vi "SpiralSearchForObserver.vi"() -> ()   [LabVIEW 2009, in "DelayGenerator.lvlib"]
uses:
  DelayGenerator.lvlib
  Aerotech/Controls/AerotechTarget.ctl
  Controls/DelayGenerator.ctl
  <vilib>/Utility/file.llb/Write To Spreadsheet File (string).vi
panel:
  out "Equivalent 0 OPD Aerotech":dbl[unit]=0.4973897187765687
  out "Actual Offset (real)":dbl[unit]=-0.9947794375531374
  in  "Tab Control":enum32{"OffSet", "Aerotech Position"}(tab)
  out "Waveform Chart":dbl[unit](graph)=-0.9947794375531374
  out "Aerotech":T1(graph)
  in  "file (use dialog)":path=path "C:/Ohana_Development/Data/Ciel juillet 2010/logOffset120710.txt"
  in  "Central Carriage\nPosition":dbl[unit]=5.4
  in  "longueur":dbl[unit]=0.000128
  out "timeout":bool
  out "AEROTECH.ACTUAL":T2={"Time"=timestamp(3360926630.935375 s since 1904-01-01), "Position"=0.49738967, "Velocity"=2.43882843364851e-08}
  in  "0 OPD Aerotech position at 5.4":dbl[unit]=0.494234
  in  "Manual step Aerotech":dbl[unit]=1.2e-05
  in  "en arrière":bool
  in  "en avant":bool
  in  "Automatic":bool
  in  "Gain":dbl=0.3
  out "amplitude mouvement":dbl[unit]=2.133333333333333e-05
  out "compteur":i32=3565
  in  "+/-1":dbl=-1.0
  out "step Aerotech":dbl[unit]=2.133333333333333e-05
  in  "sens":bool=TRUE
  in  "Unidirectionnel":bool=TRUE
  out "position frange":dbl(slide)=-0.10617897727272729 max=9.49392237e-316 scale=-1.0..1.0
  out "centre spirale":dbl[unit]=0.4973897187765687
  out "Frange":bool=TRUE
  in  "stop":bool
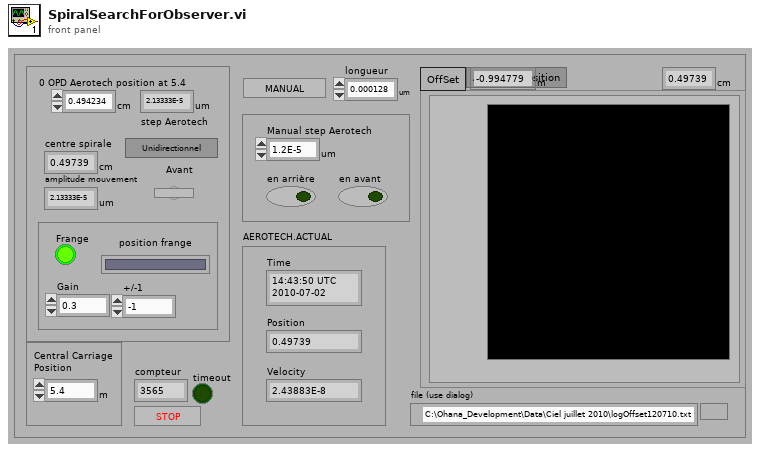
[diagram p1: front panel]
types:
  T1 = cluster{"0 OPD Aerotech position at 5.4":dbl[unit], dbl[unit]}
  T2 = typedef "AerotechTarget.ctl" = cluster{"Time":timestamp, "Position":dbl, "Velocity":dbl}
  T3 = typedef "DelayGenerator.ctl" = cluster{"OpticalPasses":i32}
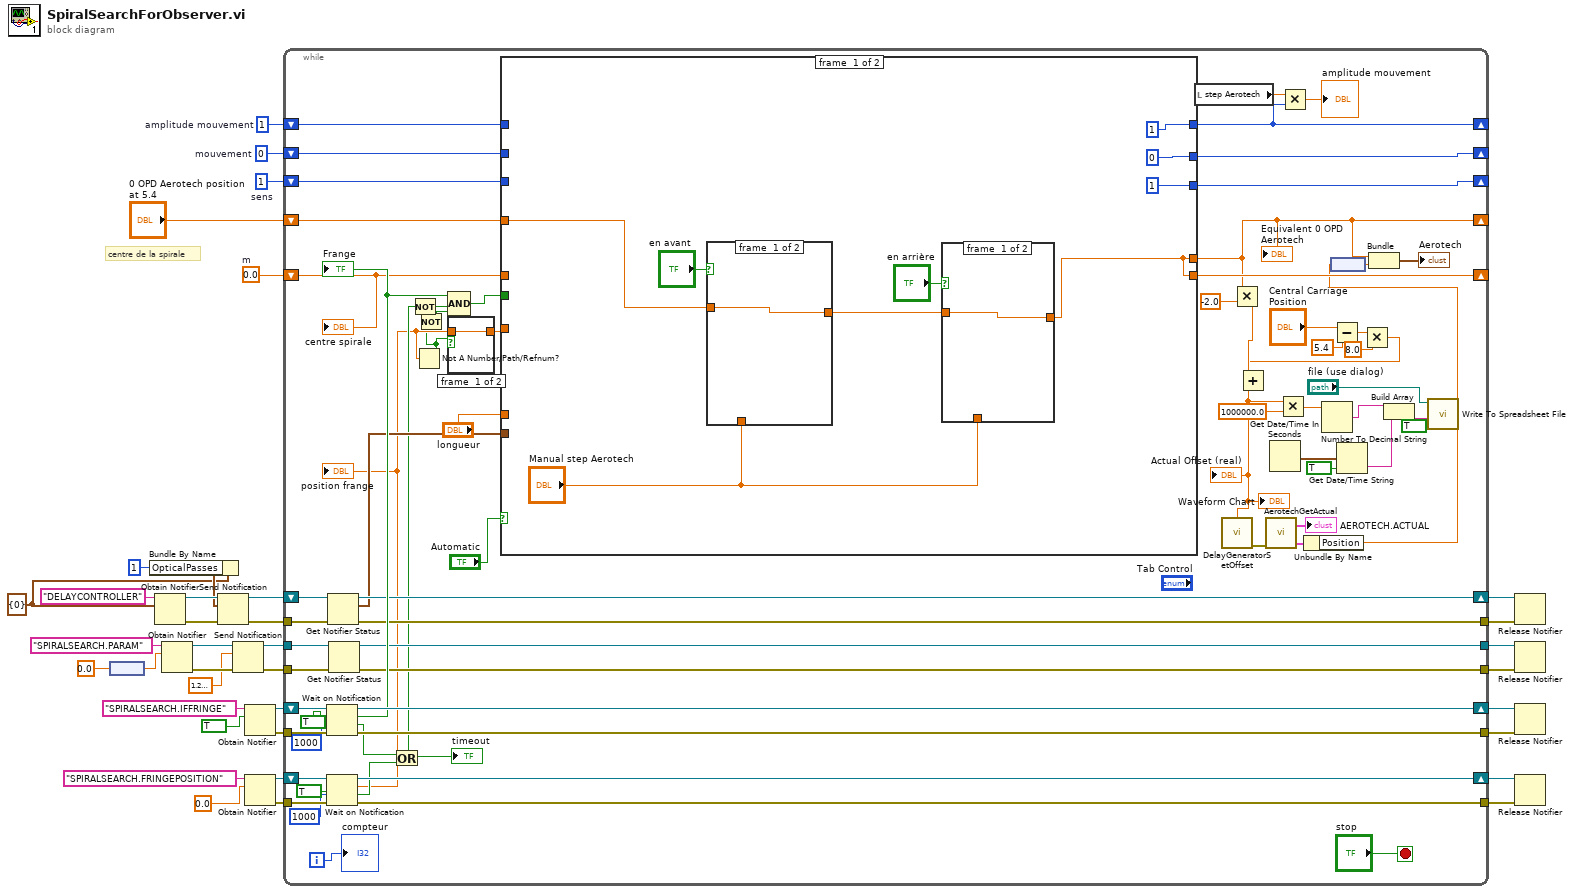
[diagram p0: block diagram]
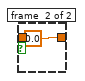
[diagram p2: hidden frame]
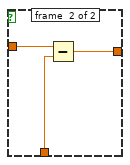
[diagram p3: hidden frame]
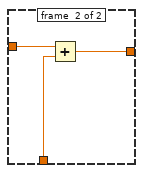
[diagram p4: hidden frame]
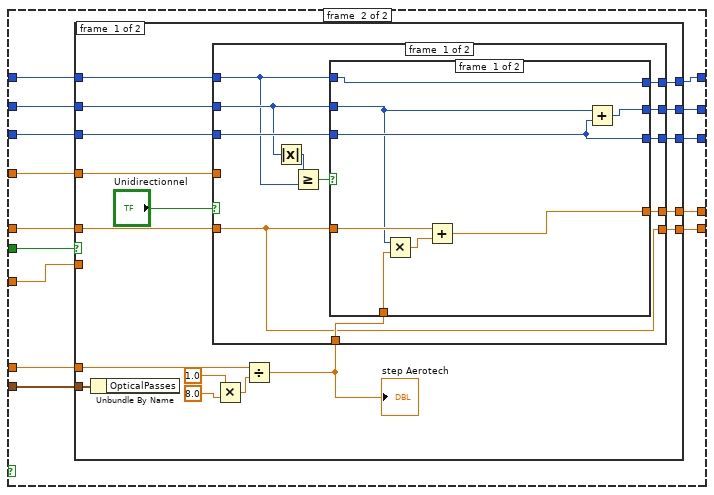
[diagram p5: hidden frame]
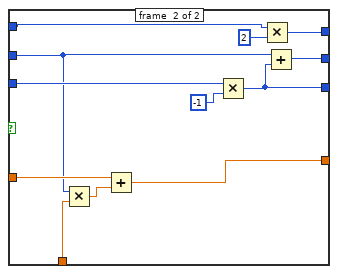
[diagram p6: hidden frame]
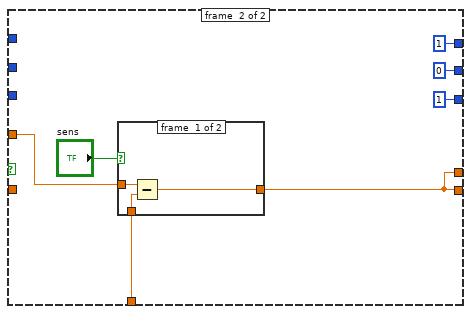
[diagram p7: hidden frame]
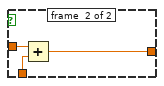
[diagram p8: hidden frame]
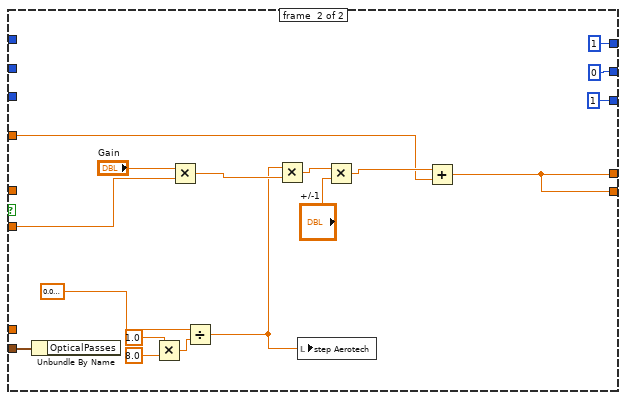
[diagram p9: hidden frame]
diagram:
  w8 = T3 {"OpticalPasses"=0} ("DelayController")
  w20 = dbl[unit] 0.0  # m
  w21 = 1  # sens
  w24 = 0  # mouvement
  w30 = 1  # amplitude mouvement
  # "centre de la spirale"
  n1 = node(0.0 ("x")) -> (w18:dbl[unit])
  n2 = Bundle By Name(cluster=w8, "OpticalPasses"=1) -> (w9:T3)
  n3 = Obtain Notifier(name (unnamed)="DELAYCONTROLLER", notification data type=w8) -> (notifier out=w15:refnum<notifier>, error out=w11:errorcluster)  [unwired: 2 in, 1 out]
  n4 = Obtain Notifier(name (unnamed)="SPIRALSEARCH.PARAM", notification data type=w18) -> (notifier out=w3:refnum<notifier>, error out=w6:errorcluster)  [unwired: 2 in, 1 out]
  n5 = Send Notification(notification=w9, notifier=w15, error in (no error)=w11) -> (notifier out=w12:refnum<notifier>, error out=w10:errorcluster)
  n6 = Send Notification(notification=dbl[unit] 1.28e-07, notifier=w3, error in (no error)=w6) -> (notifier out=w4:refnum<notifier>, error out=w5:errorcluster)
  n7 = Obtain Notifier(name (unnamed)="SPIRALSEARCH.IFFRINGE", notification data type=TRUE) -> (notifier out=w32:refnum<notifier>, error out=w29:errorcluster)  [unwired: 2 in, 1 out]
  n8 = Obtain Notifier(name (unnamed)="SPIRALSEARCH.FRINGEPOSITION", notification data type=0.0 ("x")) -> (notifier out=w35:refnum<notifier>, error out=w27:errorcluster)  [unwired: 2 in, 1 out]
  n9 = while {
    shift-right: [w105] -> w34
    shift-left: w35 -> [w106]
    shift-right: [w103] -> w31
    shift-left: w32 -> [w104]
    shift-right: [w73] -> _
    shift-left: w30 -> [w82]
    tunnel: w29 -> [w102]
    tunnel: [w101] -> w28
    tunnel: w27 -> [w100]
    tunnel: [w99] -> w26
    shift-right: [w76] -> _
    shift-left: w20 -> [w81]
    shift-right: [w92] -> _
    shift-left: w24 -> [w93]
    shift-right: [w95] -> w23
    shift-left: w12 -> [w96]
    tunnel: w10 -> [w90]
    tunnel: [w89] -> w22
    shift-right: [w91] -> _
    shift-left: w21 -> [w88]
    shift-right: [w45] -> _
    shift-left: "0 OPD Aerotech position at 5.4" -> [w84]
    tunnel: w4 -> [w80]
    tunnel: w5 -> [w79]
    tunnel: [w78] -> w14
    tunnel: [w77] -> w13
    i -> [w87]
    stop <- "stop" stop-if-true
    n10 = Wait on Notification(notifier=w104, ignore previous (F)=TRUE, timeout in ms (-1)=1000, error in (no error)=w102) -> (notifier out=w103:refnum<notifier>, notification=w97:bool, timed out?=w67:bool, error out=w101:errorcluster)
    "Frange" <- w97
    n11 = Wait on Notification(notifier=w106, ignore previous (F)=TRUE, timeout in ms (-1)=1000, error in (no error)=w100) -> (notifier out=w105:refnum<notifier>, notification=w61:dbl, timed out?=w65:bool, error out=w99:errorcluster)
    "position frange" <- w61
    n12 = Get Notifier Status(notifier=w96, error in (no error)=w90) -> (notifier out=w95:refnum<notifier>, current notification=w94:T3, error out=w89:errorcluster)  [unwired: 2 out]
    n13 = Get Notifier Status(notifier=w80, error in (no error)=w79) -> (notifier out=w78:refnum<notifier>, error out=w77:errorcluster)  [unwired: 3 out]
    n14 = Or(x=w67, y=w65) -> (x .or. y?=w66:bool)
    "timeout" <- w66
    n15 = Not(x=w66) -> (.not. x?=w68:bool)
    n16 = Not A Number/Path/Refnum?(number/path/refnum=w61) -> (NaN/Path/Refnum?=w59:bool)
    n17 = Not(x=w59) -> (.not. x?=w60:bool)
    n18 = Compound Arithmetic op=AND(w97, w68, w60) -> (w69:bool)
    n19 = case shown="True" w59 {
      tunnel: w61 -> [w107 _]
      tunnel: [w107 0.0 ("x")] -> w62
      frame #0 {
      }
      frame #1 {
      }
    }
    n20 = case shown="True" "Automatic" {
      tunnel: w69 -> [_ w139]
      tunnel: w94 -> [_ w138]
      tunnel: w81 -> [_ w137]
      tunnel: w62 -> [_ w136]
      tunnel: w93 -> [_ w135]
      tunnel: [0 w134] -> w92
      tunnel: [1 ("sens") w133] -> w91
      tunnel: w88 -> [_ w132]
      tunnel: w84 -> [w111 w131]
      tunnel: [w109 w130] -> w45
      tunnel: w82 -> [_ w129]
      tunnel: [1 ("amplitude mouvement") w128] -> w73
      tunnel: "longueur" -> [_ w127]
      tunnel: [w109 w126] -> w76
      frame #0 {
        n21 = case shown="False" "en avant" {
          tunnel: "Manual step Aerotech" -> [_ w123]
          tunnel: w111 -> [w122 w124]
          tunnel: [w122 w125] -> w110
          frame #0 {
          }
          frame #1 {
            n22 = Add(x=w124, y=w123) -> (x+y=w125:dbl[unit])
          }
        }
        n23 = case shown="False" "en arrière" {
          tunnel: "Manual step Aerotech" -> [_ w119]
          tunnel: w110 -> [w118 w121]
          tunnel: [w118 w120] -> w109
          frame #0 {
          }
          frame #1 {
            n24 = Subtract(x=w121, y=w119) -> (x-y=w120:dbl[unit])
          }
        }
      }
      frame #1 {
        n25 = case shown="True" w139 {
          tunnel: w138 -> [w156 w204]
          tunnel: w137 -> [w149 _]
          tunnel: w136 -> [_ w217]
          tunnel: [w150 w207] -> w130
          tunnel: [w153 1 ("amplitude mouvement")] -> w128
          tunnel: [w155 0 ("mouvement")] -> w134
          tunnel: w135 -> [w151 _]
          tunnel: w132 -> [w152 _]
          tunnel: [w154 1] -> w133
          tunnel: [w145 w207] -> w126
          tunnel: w131 -> [w147 w208]
          tunnel: w129 -> [w146 _]
          tunnel: w127 -> [w142 _]
          frame #0 {
            n26 = Unbundle By Name(w156) -> ()  [unwired: 1 out]
            n27 = Multiply(x=1.0, y=8.0) -> (x*y=w143:dbl)
            n28 = Divide(x=w142, y=w143) -> (x/y=w144:dbl[unit])
            "step Aerotech" <- w144
            n29 = case shown="True" "Unidirectionnel" {
              tunnel: [w166 0] -> w155
              tunnel: [w165 1 ("sens")] -> w154
              tunnel: [w164 1 ("amplitude mouvement")] -> w153
              tunnel: w152 -> [w163 _]
              tunnel: w151 -> [w162 _]
              tunnel: [w159 w188] -> w150
              tunnel: w149 -> [w158 _]
              tunnel: w144 -> [w160 w193]
              tunnel: [w158 w188] -> w145
              tunnel: w147 -> [_ w189]
              tunnel: w146 -> [w157 _]
              frame #0 {
                n30 = Absolute Value(x=w162) -> (abs(x)=w161:i32)
                n31 = Greater Or Equal?(x=w161, y=w157) -> (x >= y?=w167:bool)
                n32 = case shown="True" w167 {
                  tunnel: w162 -> [w171 w177]
                  tunnel: [w174 w182] -> w166
                  tunnel: [w173 w183] -> w165
                  tunnel: w163 -> [w173 w185]
                  tunnel: [w168 w187] -> w164
                  tunnel: w158 -> [w175 w180]
                  tunnel: w160 -> [w172 w179]
                  tunnel: [w169 w178] -> w159
                  tunnel: w157 -> [w168 w176]
                  frame #0 {
                    n33 = Multiply(x=w171, y=w172) -> (x*y=w170:dbl[unit])
                    n34 = Add(x=w175, y=w170) -> (x+y=w169:dbl[unit])
                    n35 = Add(x=w171, y=w173) -> (x+y=w174:i32)
                  }
                  frame #1 {
                    n36 = Multiply(x=w177, y=w179) -> (x*y=w181:dbl[unit])
                    n37 = Add(x=w180, y=w181) -> (x+y=w178:dbl[unit])
                    n38 = Multiply(x=w185, y=-1) -> (x*y=w183:i32)
                    n39 = Multiply(x=w176, y=2) -> (x*y=w187:i32)
                    n40 = Add(x=w177, y=w183) -> (x+y=w182:i32)
                  }
                }
              }
              frame #1 {
                n41 = case shown="False" "sens" {
                  tunnel: w189 -> [w197 w200]
                  tunnel: w193 -> [w196 w199]
                  tunnel: [w195 w198] -> w188
                  frame #0 {
                    n42 = Subtract(x=w197, y=w196) -> (x-y=w195:dbl[unit])
                  }
                  frame #1 {
                    n43 = Add(x=w200, y=w199) -> (x+y=w198:dbl[unit])
                  }
                }
              }
            }
          }
          frame #1 {
            n44 = Unbundle By Name(w204) -> ()  [unwired: 1 out]
            n45 = Multiply(x=1.0, y=8.0) -> (x*y=w206:dbl)
            n46 = Multiply(x="Gain", y=w217) -> (x*y=w215:dbl)
            n47 = Divide(x=dbl[unit] 0.000128, y=w206) -> (x/y=w202:dbl[unit])
            n48 = Multiply(x=w202, y=w215) -> (x*y=w214:dbl[unit])
            n49 = local write "step Aerotech"(w202) -> ()
            n50 = Multiply(x=w214, y="+/-1") -> (x*y=w209:dbl[unit])
            n51 = Add(x=w209, y=w208) -> (x+y=w207:dbl[unit])
          }
        }
      }
    }
    "Equivalent 0 OPD Aerotech" <- w45
    n52 = local read "step Aerotech"() -> (w74:dbl[unit])
    n53 = Multiply(x=w45, y=-2.0) -> (x*y=w56:dbl[unit])
    n54 = Get Date/Time In Seconds() -> (seconds since 1Jan1904=w40:timestamp)
    n55 = Multiply(x=w74, y=w73) -> (x*y=→"amplitude mouvement":dbl[unit])
    n56 = Subtract(x="Central Carriage\nPosition", y=dbl[unit] 5.4) -> (x-y=w55:dbl[unit])
    n57 = Get Date/Time String(seconds (now)=w40, want seconds? (F)=TRUE) -> (time string=w38:string)  [unwired: 1 in, 1 out]
    n58 = Multiply(x=w55, y=8.0) -> (x*y=w53:dbl[unit])
    n59 = Add(x=w53, y=w56) -> (x+y=w52:dbl[unit])
    "Waveform Chart" <- w52
    "Actual Offset (real)" <- w52
    n60 = call "DelayGeneratorSetOffset.vi"("Offset"=w52) -> ("error out"=w72:errorcluster)  [unwired: 8 in]
    n61 = call "AerotechGetActual.vi"("error in (no error)"=w72) -> ("AEROTECH.ACTUAL"=w47:T2)  [unwired: 3 in, 1 out]
    "AEROTECH.ACTUAL" <- w47
    n62 = Multiply(x=w52, y=dbl[unit] 1000000.0) -> (x*y=w42:dbl)
    n63 = Unbundle By Name(w47) -> ("Position"=w46:dbl)
    n64 = Number To Decimal String(number=w42) -> (decimal integer string=w41:string)  [unwired: 1 in]
    n65 = node(w46) -> (w44:dbl[unit])
    n66 = Bundle("0 OPD Aerotech position at 5.4"=w45, w44) -> (→"Aerotech":T1)  [unwired: 1 in]
    n67 = Build Array(w41, w38) -> (w49:string[])
    n68 = call-poly <vilib>:"Write To Spreadsheet File.vi"("append to file? (new file:F)"=TRUE, "1D data"=w49, "file path (dialog if empty)"="file (use dialog)") -> ()  [unwired: 5 in, 1 out]
    "centre spirale" <- w81
    "compteur" <- w87
  }
  n69 = Release Notifier(notifier=w23, error in (no error)=w22) -> ()  [unwired: 1 in, 3 out]
  n70 = Release Notifier(notifier=w14, error in (no error)=w13) -> ()  [unwired: 1 in, 3 out]
  n71 = Release Notifier(notifier=w31, error in (no error)=w28) -> ()  [unwired: 1 in, 3 out]
  n72 = Release Notifier(notifier=w34, error in (no error)=w26) -> ()  [unwired: 1 in, 3 out]
